vi "Get From Symbol Map Old.vi"(8 "error in (no error)":errorcluster, 10 "Symbol Name":string, 11 "TwinCAT ADS in":refnum<class "TwinCAT ADS.lvclass">) -> (0 "error out":errorcluster, 2 ".NET Symbol Information":refnum<k24>, 3 "TwinCAT ADS out":refnum<class "TwinCAT ADS.lvclass">)   [LabVIEW 2018]
uses:
  TwinCAT ADS.lvclass
  TwinCAT.Ads
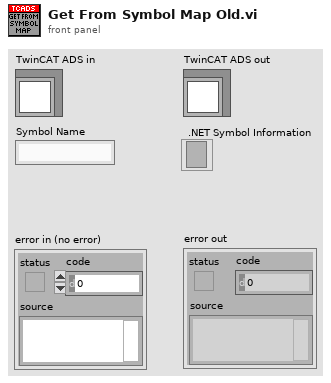
[diagram p1: front panel]
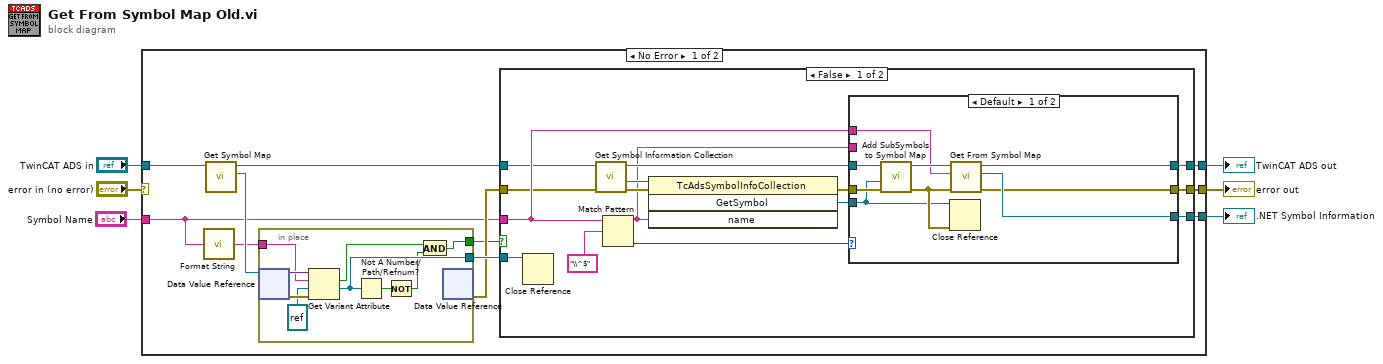
[diagram p0: block diagram]
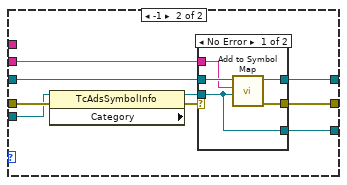
[diagram p2: hidden frame]
diagram:
  n1 = case shown="No Error" "error in (no error)" {
    selector: "error in (no error)" -> [_ w70]
    tunnel: "TwinCAT ADS in" -> [w17 w71]
    tunnel: "Symbol Name" -> [w8 _]
    tunnel: [w14 _] -> w4
    tunnel: [w10 w70] -> w3
    tunnel: [w11 w71] -> w2
    frame No Error {
      n2 = call "Format String.vi"("String"=w8) -> ("Formated String"=w7:string)
      n3 = call "Get Symbol Map.vi"("TwinCAT ADS in"=w17) -> ("Symbol Map"=w16:refnum<data-value>, "TwinCAT ADS out"=w13:refnum<class "TwinCAT ADS.lvclass">)  [unwired: 8 in, 1 out]
      n4 = in-place {
        in-place-border: w7 -> [w67]
        in-place-border: [w65] -> w15
        in-place-border: [w61] -> w9
        n5 = in-place-dvr #1(w16) -> (w68:variant, w69:errorcluster)
        n6 = Get Variant Attribute(Variant=w68, name=w67, default value (empty Variant)=refnum<k24> refnum (".NET Symbol Information"), error in=w69) -> (found=w62:bool, value=w65:refnum<k24>)  [unwired: 2 out]
        n7 = Not A Number/Path/Refnum?(number/path/refnum=w65) -> (NaN/Path/Refnum?=w64:bool)
        n8 = Not(x=w64) -> (.not. x?=w63:bool)
        n9 = And(x=w62, y=w63) -> (x .and. y?=w61:bool)
        n10 = in-place-dvr #1() -> (w12:errorcluster)  [unwired: 1 in, 1 out]
      }
      n11 = case shown="False" w9 {
        tunnel: w15 -> [w19 w60]
        tunnel: [w30 w60] -> w14
        tunnel: w8 -> [w28 _]
        tunnel: w13 -> [w21 w59]
        tunnel: w12 -> [w20 w58]
        tunnel: [w32 w59] -> w11
        tunnel: [w31 w58] -> w10
        frame False {
          n12 = Close Reference(reference=w19) -> ()  [unwired: 1 in, 1 out]
          n13 = call "Get Symbol Information Collection.vi"("error in (no error)"=w20, "TwinCAT ADS in"=w21) -> ("error out"=w27:errorcluster, ".NET AdsSymbolInfoCollection"=w26:refnum<k24>, "TwinCAT ADS out"=w24:refnum<class "TwinCAT ADS.lvclass">)  [unwired: 7 in]
          n14 = Match Pattern(string=w28, regular expression="\\^$") -> (before substring=w23:string, offset past match=w29:i32)  [unwired: 1 in, 2 out]
          n15 = invoke class="TcAdsSymbolInfoCollection" method="GetSymbol"(reference=w26, error in=w27, "name"=w23) -> (error out=w22:errorcluster, "GetSymbol"=w25:refnum<k24>)  [unwired: 1 in, 2 out]
          n16 = case shown="Default" w29 {
            tunnel: w24 -> [w40 w50]
            tunnel: [w36 w49] -> w32
            tunnel: [w33 w48] -> w31
            tunnel: [w35 w47] -> w30
            tunnel: w23 -> [_ w46]
            tunnel: w22 -> [w39 w45]
            tunnel: w25 -> [w34 w44]
            tunnel: w28 -> [w37 _]
            frame Default {
              n17 = call "Add SubSymbols to Symbol Map.vi"("error in (no error)"=w39, ".NET TcAdsSymbolInfo"=w34, "TwinCAT ADS in"=w40) -> ("error out"=w41:errorcluster, "TwinCAT ADS out"=w38:refnum<class "TwinCAT ADS.lvclass">)  [unwired: 7 in]
              n18 = Close Reference(reference=w34, error in (no error)=w41) -> ()  [unwired: 1 out]
              n19 = call "Get From Symbol Map.vi"("error in (no error)"=w41, "Symbol Name"=w37, "TwinCAT ADS in"=w38) -> ("error out"=w33:errorcluster, ".NET Symbol Information"=w35:refnum<k24>, "TwinCAT ADS out"=w36:refnum<class "TwinCAT ADS.lvclass">)  [unwired: 6 in]
            }
            frame -1 {
              n20 = property class="TcAdsSymbolInfo" props=["Category"](reference=w44, error in=w45) -> (reference out=w42:refnum<k24>, error out=w43:errorcluster)  [unwired: 1 out]
              n21 = case shown="No Error" w43 {
                selector: w43 -> [_ w57]
                tunnel: w42 -> [w51 _]
                tunnel: w50 -> [w55 w56]
                tunnel: [w54 w56] -> w49
                tunnel: w46 -> [w53 _]
                tunnel: [w52 w57] -> w48
                tunnel: [w51 _] -> w47
                frame No Error {
                  n22 = call "Add to Symbol Map.vi"(".NET Symbol Information"=w51, "Symbol Name"=w53, "TwinCAT ADS in"=w55) -> ("error out"=w52:errorcluster, "TwinCAT ADS out"=w54:refnum<class "TwinCAT ADS.lvclass">)  [unwired: 6 in, 1 out]
                }
                frame Error {
                }
              }
            }
          }
        }
        frame True {
        }
      }
    }
    frame Error {
    }
  }
  "error out" <- w3
  "TwinCAT ADS out" <- w2
  ".NET Symbol Information" <- w4
